vi "Inline or forked test handler.vi"() -> ()   [LabVIEW 2017]
uses:
  Plugins/Utility/Inline or Forked.ctl
  <vilib>/Utility/traverseref.llb/TRef TravTarget.ctl
  <vilib>/Utility/miscctls.llb/LVPointTypeDef.ctl
panel:
  in  "Inline or Forked":T1
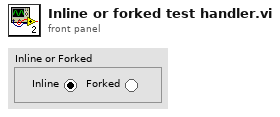
[diagram p1: front panel]
types:
  T1 = typedef "Inline or Forked.ctl" = enum32{"Inline", "Forked"}
  T2 = typedef "LVPointTypeDef.ctl" = cluster{"Horizontal":i16, "Vertical":i16}
  T3 = typedef "TRef TravTarget.ctl" = enum16{"FP", "BD", "Other"}
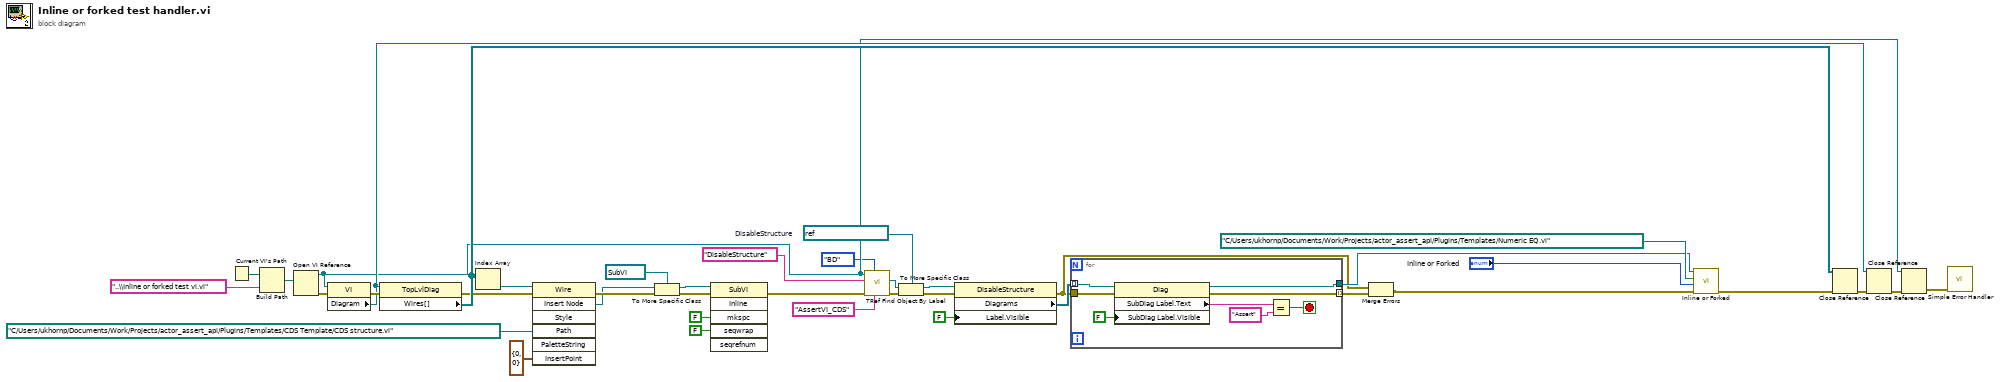
[diagram p0: block diagram]
diagram:
  w13 = refnum<vi> refnum  # DisableStructure
  n1 = Current VI's Path() -> (path=w40:path)
  n2 = Build Path(base path=w40, name or relative path="..\\Inline or forked test vi.vi") -> (appended path=w38:path)
  n3 = Open VI Reference(vi path=w38) -> (vi reference=w18:refnum<vi>, error out=w37:errorcluster)  [unwired: 5 in]
  n4 = property class="VI"(reference=w18, error in=w37) -> (error out=w36:errorcluster, "Diagram"=w35:refnum<vi>)  [unwired: 1 out]
  n5 = property class="TopLvlDiag"(reference=w35, error in=w36) -> (error out=w30:errorcluster, "Wires[]"=w32:refnum<vi>[])  [unwired: 1 out]
  n6 = Index Array(array=w32) -> (element=w28:refnum<vi>)  [unwired: 1 in]
  n7 = invoke class="Wire" method="Insert Node"(reference=w28, error in=w30, "Path"=path "C:/Users/ukhornp/Documents/Work/Projects/actor_assert_api/Plugins/Templates/CDS Template/CDS structure.vi", "InsertPoint"=T2 {"Horizontal"=0, "Vertical"=0} ("Insertion Point")) -> (error out=w29:errorcluster, "Insert Node"=w26:refnum<vi>)  [unwired: 3 in, 5 out]
  n8 = To More Specific Class(target class=refnum<vi> refnum ("reference"), reference=w26, error in=w29) -> (specific class reference=w24:refnum<vi>, error out=w21:errorcluster)
  n9 = invoke class="SubVI" method="Inline"(reference=w24, error in=w21, "mkspc"=FALSE ("Make Space in Block Diagram"), "seqwrap"=FALSE ("Wrap in Sequence")) -> (error out=w20:errorcluster)  [unwired: 2 in, 5 out]
  n10 = call <vilib>:"TRef Find Object By Label.vi"("Label"="AssertVI_CDS", "Traverse Target"=TRef_TravTarget."BD", "error in (no error)"=w20, "Class Name"="DisableStructure", "VI Ref"=w18) -> ("error out"=w19:errorcluster, "Found Obj Ref"=w14:refnum<vi>)  [unwired: 3 in, 2 out]
  n11 = To More Specific Class(target class=w13, reference=w14, error in=w19) -> (specific class reference=w12:refnum<vi>, error out=w11:errorcluster)
  n12 = property class="DisableStructure"(reference=w12, error in=w11, "Label.Visible"=FALSE) -> (error out=w2:errorcluster, "Diagrams"=w10:refnum<vi>[])  [unwired: 1 out]
  n13 = for {
    tunnel: w10 -> [w48] mode=indexing
    tunnel: [w44] -> w4
    tunnel: w2 -> [w42]
    tunnel: [w41] -> w9 mode=indexing
    stop <- w45 stop-if-true
    n14 = property class="Diag"(reference=w48, error in=w42, "SubDiag Label.Visible"=FALSE ("Subdiagram Label.Visible")) -> (reference out=w44:refnum<vi>, error out=w41:errorcluster, "SubDiag Label.Text"=w47:string)
    n15 = Equal?(x=w47, y="Assert") -> (x = y?=w45:bool)
  }
  n16 = Merge Errors(w2, w9) -> (w3:errorcluster)
  n17 = call "Inline or Forked.vi"("error in (no error)"=w3, "Inline or Forked"="Inline or Forked", "Assert VI Path"=path "C:/Users/ukhornp/Documents/Work/Projects/actor_assert_api/Plugins/Templates/Numeric EQ.vi", "Diagram in"=w4) -> ("error out"=w1:errorcluster)  [unwired: 7 in]
  n18 = Close Reference(reference=w32, error in (no error)=w1) -> (error out=w34:errorcluster)
  n19 = Close Reference(reference=w35, error in (no error)=w34) -> (error out=w33:errorcluster)
  n20 = Close Reference(reference=w18, error in (no error)=w33) -> (error out=w5:errorcluster)
  n21 = call <vilib>:"Simple Error Handler.vi"("error in (no error)"=w5) -> ()  [unwired: 4 in, 5 out]
